vi "Monitor VI Position - Async..vi"(11 "VI ref.":refnum<vi>) -> ()   [LabVIEW 2019, in "Window Mover.lvlib"]
doc: "This VI enables panel click-drag behavior on a borderless window. This is an asynchronous VI that will run in the background until the monitored VI stops running.\n\nYou must provide a VI reference to the VI you wish to monitor."
uses:
  Window Mover.lvlib
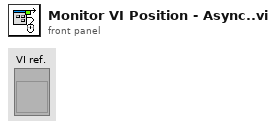
[diagram p1: front panel]
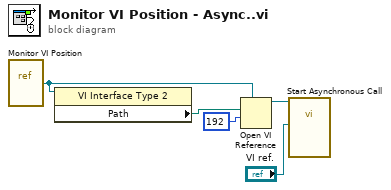
[diagram p0: block diagram]
diagram:
  n1 = vi-ref "Monitor VI Position.vi"() -> (w2:refnum<vi>)
  n2 = property class="VI Interface Type 2"(reference=w2) -> ("Path"=w5:path)  [unwired: 1 in, 2 out]
  n3 = Open VI Reference(type specifier VI Refnum (for type only)=w2, vi path=w5, options=192) -> (vi reference=w3:refnum<vi>)  [unwired: 3 in, 1 out]
  n4 = call-by-ref "Start Asynchronous Call"(reference=w3, "VI ref."="VI ref.") -> ()  [unwired: 12 in, 2 out]
